vi "WS1021 Stress Beams.vi"(8 "error in (no error)":errorcluster, 11 "Cycling Bit":string[](array[string])=["0701020303", "0701020000"]) -> (0 "error out":errorcluster, 2 "Cmd":string, 3 "Beams":string)   [LabVIEW 2017]
uses:
  <vilib>/Utility/error.llb/whitespace.ctl
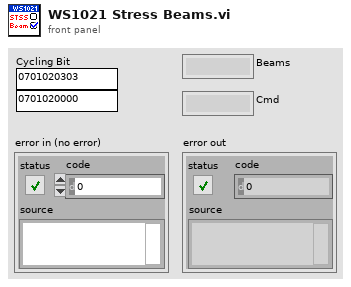
[diagram p1: front panel]
types:
  T1 = typedef "whitespace.ctl" = u16
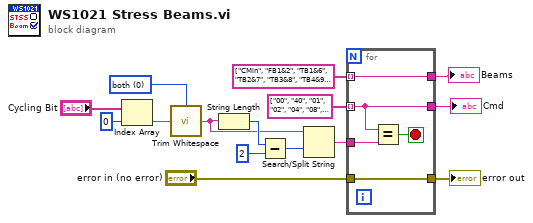
[diagram p0: block diagram]
diagram:
  w12 = T1 0 items=["both", "start of string", "end of string"] ("location (both)")
  n1 = Index Array(array="Cycling Bit", index=0) -> (element=w13:string)
  n2 = call <vilib>:"Trim Whitespace.vi"("string"=w13, "location (both)"=w12) -> ("trimmed string"=w8:string)
  n3 = String Length(string=w8) -> (length=w11:i32)
  n4 = Subtract(x=w11, y=2) -> (x-y=w9:i32)
  n5 = Search/Split String(string=w8, offset (0)=w9) -> (match + rest of string=w7:string)  [unwired: 1 in, 2 out]
  n6 = for {
    tunnel: w7 -> [w20]
    tunnel: string[] ["00", "40", "01", "02", "04", "08", "10", "20", "7F"] -> [w18] mode=indexing
    tunnel: [w18] -> w3
    tunnel: string[] ["CMin", "FB1&2", "TB1&6", "TB2&7", "TB3&8", "TB4&9", "TB5&10", "TB3&TB11", "ALL"] -> [w17] mode=indexing
    tunnel: [w17] -> w4
    tunnel: "error in (no error)" -> [w16]
    tunnel: [w16] -> w1
    stop <- w19 stop-if-true
    n7 = Equal?(x=w18, y=w20) -> (x = y?=w19:bool)
  }
  "Beams" <- w4
  "Cmd" <- w3
  "error out" <- w1
